vi "testClearConstantError.vi"(8 "error in (no error)":errorcluster, 11 "TestCase in":refnum<class "Data Manipulation Tests.lvclass">) -> (0 "error out":errorcluster, 3 "TestCase out":refnum<class "Data Manipulation Tests.lvclass">)   [LabVIEW 2017, in "Pointer Tests.lvlib" / "Data Manipulation Tests.lvclass"]
uses:
  Data Manipulation Tests.lvclass
  Source/Classes/Pointer/Public/New/New (1B).vi
  Source/Classes/Pointer/Public/Write/Write (0D U8).vi
  Source/Classes/Pointer/Public/Read/Read (0D U8).vi
  <vilib>/addons/_JKI Toolkits/VI Tester/TestCase.llb/TestCase.lvclass
  Source/Classes/Pointer/Pointer.lvclass
  C:/Program Files (x86)/National Instruments/LabVIEW 2017/vi.lib/addons/_JKI Toolkits/VI Tester/TestCase.llb/TestCase.lvclass
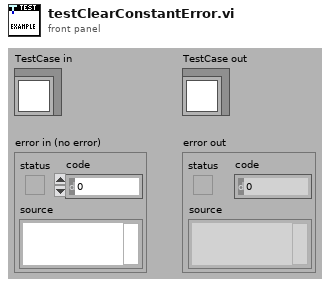
[diagram p1: front panel]
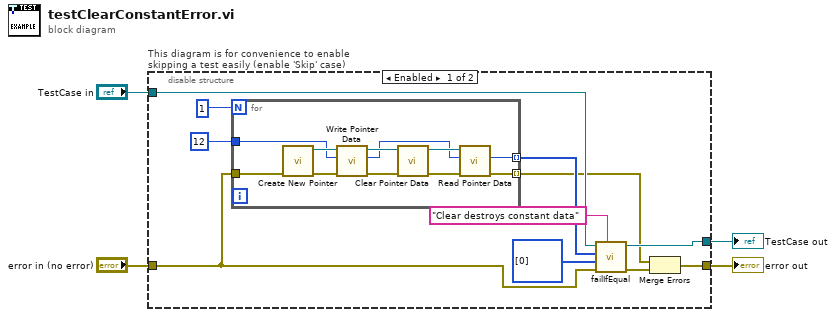
[diagram p0: block diagram]
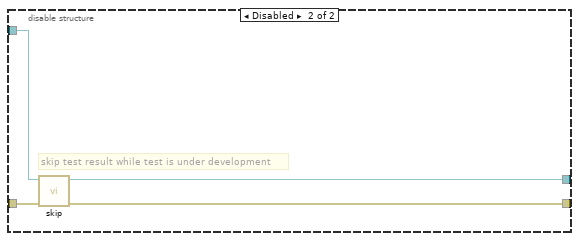
[diagram p2: hidden frame]
diagram:
  n1 = disable-structure "This diagram is for convenience to enable skipping a test easily (enable 'Skip' case)" shown="Enabled" {
    disable-tunnel: "TestCase in" -> [w15 w30]
    disable-tunnel: [w13 w28] -> w1
    disable-tunnel: [w7 w29] -> w3
    disable-tunnel: "error in (no error)" -> [w6 w27]
    frame Enabled {
      n2 = for {
        N: 1 -> [_]
        tunnel: w6 -> [w26]
        tunnel: [w18] -> w11 mode=indexing
        tunnel: u8 12 -> [w17]
        tunnel: [w16] -> w9 mode=indexing
        n3 = call-poly "Create New Pointer.vi"("error in (no error)"=w26) -> ("error out"=w20:errorcluster, "Pointer"=w21:refnum<class "Pointer.lvclass">)  [unwired: 9 in]
        n4 = call-poly "Write Pointer Data.vi"("error in (no error)"=w20, "value"=w17, "Pointer in"=w21) -> ("error out"=w24:errorcluster, "value"=w19:u8, "Pointer out"=w25:refnum<class "Pointer.lvclass">)  [unwired: 5 in, 1 out]
        n5 = call "Clear Pointer Data.vi"("error in (no error)"=w24, "Pointer in"=w25) -> ("error out"=w22:errorcluster, "Pointer out"=w23:refnum<class "Pointer.lvclass">)  [unwired: 8 in]
        n6 = call-poly "Read Pointer Data.vi"("error in (no error)"=w22, "value in"=w19, "Pointer in"=w23) -> ("error out"=w16:errorcluster, "value out"=w18:u8)  [unwired: 5 in, 2 out]
      }
      n7 = call-dynamic "failIfEqual.vi"("custom report message (\"\")"="Clear destroys constant data" ("custom report message (\"\")"), "error in (no error)"=w6, "y"=u8[] [0] ("Array"), "x"=w11, "TestCase in"=w15) -> ("error out"=w8:errorcluster, "TestCase out"=w13:refnum<class "Data Manipulation Tests.lvclass">)  [unwired: 5 in]
      n8 = Merge Errors(w9, w8) -> (w7:errorcluster)
    }
    frame Disabled {
      # "skip test result while test is under development"
      n9 = call <vilib>:"skip.vi"("error in (no error)"=w27, "TestCase in"=w30) -> ("error out"=w29:errorcluster, "TestCase out"=w28:refnum<class "Data Manipulation Tests.lvclass">)  [unwired: 8 in]
    }
  }
  "error out" <- w3
  "TestCase out" <- w1
